vi "SMO.UI.TestLauncher.vi"() -> ()   [LabVIEW 2013, in "SMO.UI.lvclass"]
uses:
  SMO.UI.lvclass
  SMO/SMO.lvclass
panel:
  out "error out":errorcluster
  in  "Stop":bool
  # "SMO.UI Test Launcher"
  # "For instructions on how to use the JKI State Machine Objects, examples and video tutorials, visit:\nhttp://jki.net/state-machine-objects/\n\nJKI State Machine Objects™\nhttp://jki.net/state-machine-objects/\nCopyright (C) 2005-2015, JKI <info@jki.net>\nALL RIGHTS RESERVED"
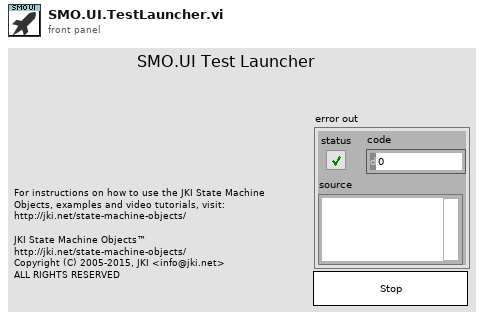
[diagram p1: front panel]
types:
  T1 = cluster{"SMO.UI Public Events":refnum<event-registration>}
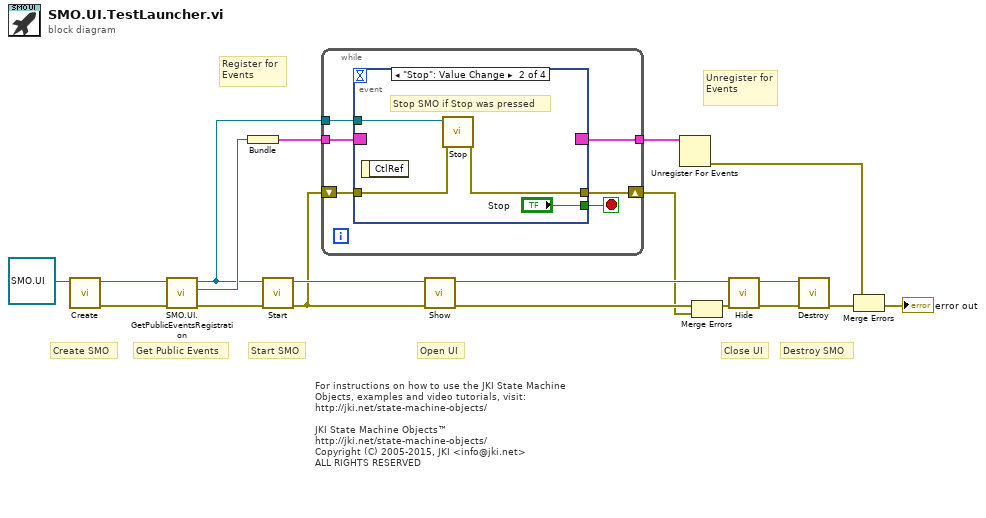
[diagram p0: block diagram]
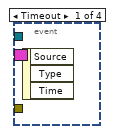
[diagram p2: hidden frame]
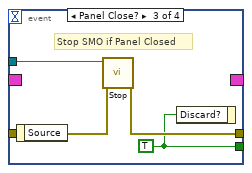
[diagram p3: hidden frame]
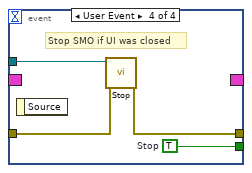
[diagram p4: hidden frame]
diagram:
  # "For instructions on how to use the JKI State Machine Objects, examples and video tutorials, visit:\nhttp://jki.net/state-machine-objects/\n\nJKI State Machine Objects™\nhttp://jki.net/state-machine-objects/\nCopyright (C) 2005-2015, JKI <info@jki.net>\nALL RIGHTS RESERVED"
  # "Get Public Events"
  # "Start SMO"
  # "Destroy SMO"
  # "Create SMO"
  # "Close UI"
  # "Open UI"
  # "Unregister for Events"
  # "Register for Events"
  n1 = call "Create.vi"("SMO"=refnum<class "SMO.UI.lvclass"> refnum ("SMO.UI.lvclass")) -> ("error out"=w7:errorcluster, "SMO out"=w8:refnum<class "SMO.UI.lvclass">)  [unwired: 9 in]
  n2 = call "SMO.UI.GetPublicEventsRegistration.vi"("error in (no error)"=w7, "SMO.UI"=w8) -> ("error out"=w18:errorcluster, "SMO.UI Public Events"=w17:refnum<event-registration>, "SMO.UI out"=w4:refnum<class "SMO.UI.lvclass">)  [unwired: 7 in]
  n3 = Bundle("SMO.UI Public Events"=w17) -> (w16:T1)  [unwired: 1 in]
  n4 = call "Start.vi"("error in (no error)"=w18, "SMO"=w4) -> ("error out"=w6:errorcluster, "SMO out"=w15:refnum<class "SMO.UI.lvclass">)  [unwired: 8 in]
  n5 = while {
    shift-right: [w24] -> w5
    shift-left: w6 -> [w23]
    tunnel: w16 -> [w22]
    tunnel: [w21] -> w19
    tunnel: w4 -> [w20]
    stop <- w25 stop-if-true
    n6 = event shown="[1] \"Stop\": Value Change" {
      selector: w22 -> [_ _ _ _]
      dyn-events: [_ _ _ _] -> w21
      timeout: _ -> [_ _ _ _]
      tunnel: [_ "Stop" w30 w34] -> w25
      tunnel: w20 -> [_ w28 w33 w37]
      tunnel: [_ w27 w32 w36] -> w24
      tunnel: w23 -> [_ w26 w31 w35]
      event Timeout {
        n7 = event-data() -> ()  [unwired: 1 in, 3 out]
      }
      event "Stop": Value Change {
        # "Stop SMO if Stop was pressed"
        n8 = event-data() -> ()  [unwired: 1 in, 1 out]
        n9 = call "Stop.vi"("error in (no error)"=w26, "SMO"=w28) -> ("error out"=w27:errorcluster)  [unwired: 8 in, 1 out]
      }
      event Panel Close? {
        w30 = TRUE ("OK")
        # "Stop SMO if Panel Closed"
        n10 = event-data() -> ()  [unwired: 1 in, 1 out]
        n11 = call "Stop.vi"("error in (no error)"=w31, "SMO"=w33) -> ("error out"=w32:errorcluster)  [unwired: 8 in, 1 out]
        n12 = event-data("Discard?"=w30) -> ()  [unwired: 1 in, 1 out]
      }
      event User Event {
        w34 = TRUE  # Stop
        # "Stop SMO if UI was closed"
        n13 = event-data() -> ()  [unwired: 1 in, 1 out]
        n14 = call "Stop.vi"("error in (no error)"=w35, "SMO"=w37) -> ("error out"=w36:errorcluster)  [unwired: 8 in, 1 out]
      }
    }
  }
  n15 = call "Show.vi"("error in (no error)"=w6, "SMO.UI"=w15) -> ("error out"=w14:errorcluster, "SMO.UI out"=w13:refnum<class "SMO.UI.lvclass">)  [unwired: 8 in]
  n16 = Unregister For Events(event registration refnum=w19) -> (error out=w3:errorcluster)  [unwired: 1 in]
  n17 = Merge Errors(w14, w5) -> (w11:errorcluster)
  n18 = call "Hide.vi"("error in (no error)"=w11, "SMO.UI"=w13) -> ("error out"=w10:errorcluster, "SMO.UI out"=w12:refnum<class "SMO.UI.lvclass">)  [unwired: 8 in]
  n19 = call "Destroy.vi"("error in (no error)"=w10, "SMO"=w12) -> ("error out"=w1:errorcluster)  [unwired: 9 in]
  n20 = Merge Errors(w3, w1) -> (→"error out":errorcluster)
